vi "Unreserve (N Sessions).vi"(8 "error in":errorcluster, 10 "session information":T3[](array[typedef]), 11 "gRPC clients":T1) -> (0 "error out":errorcluster)   [LabVIEW 2020, in "Measurement Service Helpers.lvlib"]
doc: "Unreserves the sessions based on the given session information."
uses:
  Measurement Service Helpers.lvlib
  <vilib>/MeasurementLink/MeasurementLink Session Management Client/RPC Messages/ni_measurementlink_sessionmanagement_v1_SessionInformation.ctl
  <vilib>/MeasurementLink/MeasurementLink Session Management Client/RPC Messages/nidevice_grpc_Session.ctl
  <vilib>/MeasurementLink/MeasurementLink Session Management Client/RPC Messages/ni_measurementlink_sessionmanagement_v1_ChannelMapping.ctl
  GRPC Clients.ctl
  <vilib>/gRPC/LabVIEW gRPC Library/Shared/grpcId.ctl
  <vilib>/MeasurementLink/MeasurementLink Session Management Client/RPC Messages/ni_measurementlink_sessionmanagement_v1_UnreserveSessionsRequest.ctl
  <vilib>/MeasurementLink/MeasurementLink Discovery Client/MeasurementLink Discovery Client.lvlib
  <vilib>/MeasurementLink/MeasurementLink Session Management Client/MeasurementLink Session Management Client.lvlib
  <vilib>/gRPC/LabVIEW gRPC Library/grpc-lvsupport-release.lvlib
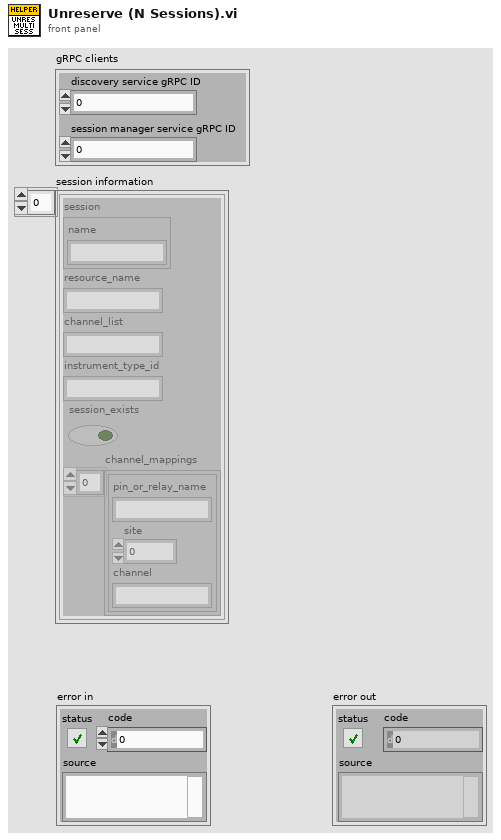
[diagram p1: front panel]
types:
  T1 = typedef "Measurement Service Helpers.lvlib/GRPC Clients.ctl" = cluster{"discovery service gRPC ID":T2, "session manager service gRPC ID":T2}
  T2 = typedef "grpc-lvsupport-release.lvlib/grpcId.ctl" = u64
  T3 = typedef "MeasurementLink Session Management Client.lvlib/ni_measurementlink_sessionmanagement_v1_SessionInformation.ctl" = cluster{"session":T4, "resource_name":string, "channel_list":string, "instrument_type_id":string, "session_exists":bool, "channel_mappings":T5[]}
  T4 = typedef "MeasurementLink Session Management Client.lvlib/nidevice_grpc_Session.ctl" = cluster{"name":string}
  T5 = typedef "MeasurementLink Session Management Client.lvlib/ni_measurementlink_sessionmanagement_v1_ChannelMapping.ctl" = cluster{"pin_or_relay_name":string, "site":i32, "channel":string}
  T6 = typedef "MeasurementLink Session Management Client.lvlib/ni_measurementlink_sessionmanagement_v1_UnreserveSessionsRequest.ctl" = cluster{"sessions":T3[]}
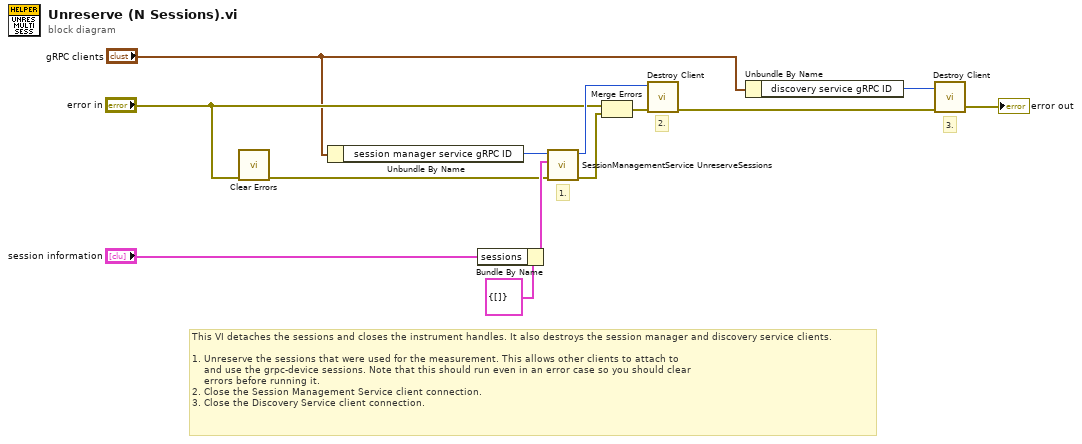
[diagram p0: block diagram]
diagram:
  # "This VI detaches the sessions and closes the instrument handles. It also destroys the session manager and discovery service clients.\n\n1. Unreserve the sessions that were used for the measurement. This allows other clients to attach to\n    and use the grpc-device sessions. Note that this should run even in an error case so you should clear \n    errors before running it.\n2. Close the Session Management Service client connection.\n3. Close the Discovery Service client connection."
  # "1."
  # "3."
  # "2."
  n1 = call <vilib>:"Clear Errors.vi"("error in (no error)"="error in") -> ("error out"=w4:errorcluster)  [unwired: 5 in, 1 out]
  n2 = Unbundle By Name("gRPC clients") -> ("session manager service gRPC ID"=w3:T2)
  n3 = Bundle By Name(cluster=T6 {"sessions"=[]} ("Request Data"), "sessions"="session information") -> (w10:T6)
  n4 = call <vilib>:"SessionManagementService UnreserveSessions.vi"("error in"=w4, "Request Data"=w10, "gRPC ID"=w3) -> ("error out"=w8:errorcluster, "gRPC ID out"=w13:T2)  [unwired: 6 in, 1 out]
  n5 = Merge Errors("error in", w8) -> (w9:errorcluster)
  n6 = call <vilib>:"Destroy Client.vi"("error in"=w9, "gRPC ID"=w13) -> ("error out"=w12:errorcluster)  [unwired: 9 in]
  n7 = Unbundle By Name("gRPC clients") -> ("discovery service gRPC ID"=w2:T2)
  n8 = call <vilib>:"Destroy Client.vi"("error in"=w12, "gRPC ID"=w2) -> ("error out"=→"error out":errorcluster)  [unwired: 9 in]
